vi "FindNodeByID.vi"(8 "error in (no error)":errorcluster, 9 "Node ID":string="//rect", 10 "Node Name (exact)":string="//rect", 11 "ParseSVG in":refnum<class "ParseSVG.lvclass">) -> (0 "error out":errorcluster, 2 "ID Match Node":refnum<k20>, 3 "ParseSVG out":refnum<class "ParseSVG.lvclass">)   [LabVIEW 2019, in "ParseSVG.lvclass"]
uses:
  ParseSVG.lvclass
  <vilib>/xml/NI_XML.lvlib
  <vilib>/xml/Close Reference(Node).vi
  <resource>/objmgr/DOMUserDefRef.rc
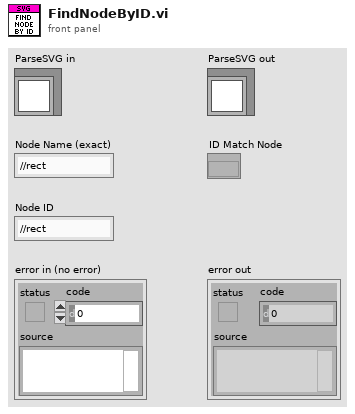
[diagram p1: front panel]
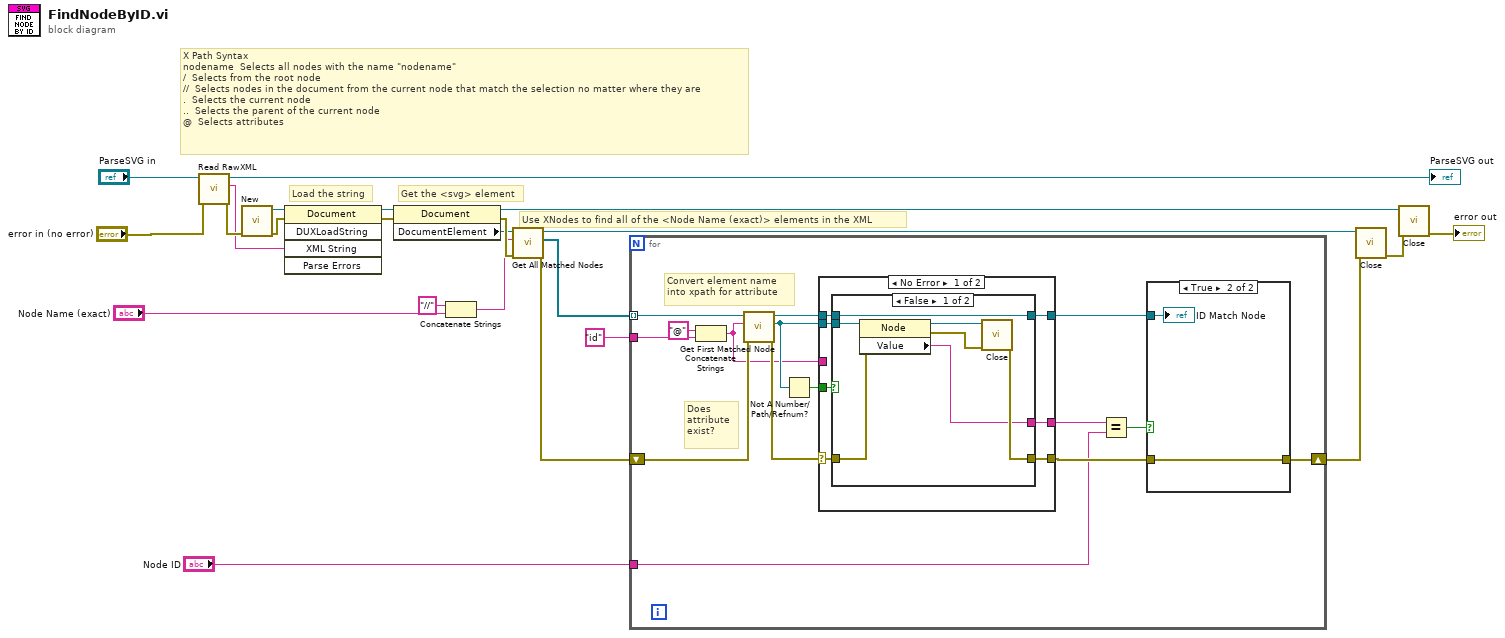
[diagram p0: block diagram]
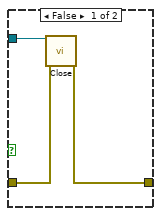
[diagram p2: hidden frame]
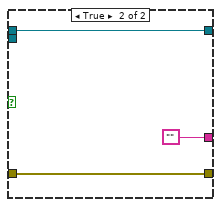
[diagram p3: hidden frame]
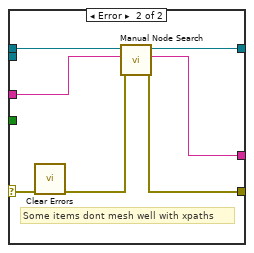
[diagram p4: hidden frame]
diagram:
  # "X Path Syntax\nnodename \tSelects all nodes with the name \"nodename\"\n/ \tSelects from the root node\n// \tSelects nodes in the document from the current node that match the selection no matter where they are\n. \tSelects the current node\n.. \tSelects the parent of the current node\n@ \tSelects attributes"
  # "Use XNodes to find all of the <Node Name (exact)> elements in the XML"
  # "Get the <svg> element"
  # "Load the string"
  n1 = call "Read RawXML.vi"("error in (no error)"="error in (no error)", "ParseXML in"="ParseSVG in") -> ("error out"=w22:errorcluster, "RawXML"=w8:string, "ParseXML out"=→"ParseSVG out":refnum<class "ParseSVG.lvclass">)  [unwired: 7 in]
  n2 = call <vilib>:"New.vi"("error in (no error)"=w22) -> ("error out"=w21:errorcluster, "DOM document out"=w17:refnum<k20>)  [unwired: 7 in]
  n3 = invoke class="Document" method="DUXLoadString"(reference=w17, error in=w21, "XML String"=w8) -> (reference out=w16:refnum<k20>, error out=w20:errorcluster)  [unwired: 2 in, 3 out]
  n4 = property class="Document"(reference=w16, error in=w20) -> (reference out=w15:refnum<k20>, error out=w19:errorcluster, "DocumentElement"=w14:refnum<k20>)
  n5 = Concatenate Strings("//" ("string"), "Node Name (exact)") -> (w10:string)
  n6 = call <vilib>:"Get All Matched Nodes.vi"("error in (no error)"=w19, "XPath expression"=w10, "node in"=w14) -> ("error out"=w2:errorcluster, "node result array"=w12:refnum<k20>[], "node out"=w13:refnum<k20>)  [unwired: 6 in]
  n7 = for {
    tunnel: w12 -> [w36] mode=indexing
    shift-right: [w34] -> w23
    shift-left: w2 -> [w37]
    tunnel: "id" -> [w33]
    tunnel: "Node ID" -> [w25]
    # "Convert element name into xpath for attribute"
    # "Does attribute exist?"
    n8 = Concatenate Strings("@" ("string"), w33) -> (w27:string)
    n9 = call <vilib>:"Get First Matched Node.vi"("error in (no error)"=w37, "XPath expression"=w27, "node in"=w36) -> ("error out"=w32:errorcluster, "node result"=w31:refnum<k20>, "node out"=w29:refnum<k20>)  [unwired: 6 in]
    n10 = Not A Number/Path/Refnum?(number/path/refnum=w31) -> (NaN/Path/Refnum?=w30:bool)
    n11 = case shown="No Error" w32 {
      selector: w32 -> [w49 w66]
      tunnel: [w50 w67] -> w38
      tunnel: w31 -> [w48 _]
      tunnel: w30 -> [w47 _]
      tunnel: w29 -> [w46 w63]
      tunnel: [w45 w64] -> w35
      tunnel: [w44 w61] -> w26
      tunnel: w27 -> [_ w62]
      frame No Error {
        n12 = case shown="False" w47 {
          tunnel: w49 -> [w57 w60]
          tunnel: [w56 w60] -> w50
          tunnel: w48 -> [w54 _]
          tunnel: w46 -> [w53 w59]
          tunnel: [w53 w59] -> w45
          tunnel: [w52 ""] -> w44
          frame False {
            n13 = property class="Node"(reference=w54, error in=w57) -> (reference out=w55:refnum<k20>, error out=w51:errorcluster, "Value"=w52:string)
            n14 = call-poly <vilib>:"Close.vi"("error in (no error)"=w51, "node"=w55) -> ("error out"=w56:errorcluster)  [unwired: 7 in]
          }
          frame True {
          }
        }
      }
      frame Error {
        # "Some items dont mesh well with xpaths"
        n15 = call <vilib>:"Clear Errors.vi"("error in (no error)"=w66) -> ("error out"=w65:errorcluster)  [unwired: 5 in, 1 out]
        n16 = call "Manual Node Search.vi"("error in (no error)"=w65, "XPath Syntax"=w62, "Node in"=w63) -> ("error out"=w67:errorcluster, "Value"=w61:string, "Node out"=w64:refnum<k20>)  [unwired: 6 in]
      }
    }
    n17 = Equal?(x=w26, y=w25) -> (x = y?=w24:bool)
    n18 = case shown="True" w24 {
      tunnel: w38 -> [w40 w43]
      tunnel: w35 -> [w41 w42]
      tunnel: [w39 w43] -> w34
      frame False {
        n19 = call-poly <vilib>:"Close.vi"("error in (no error)"=w40, "node"=w41) -> ("error out"=w39:errorcluster)  [unwired: 7 in]
      }
      frame True {
        "ID Match Node" <- w42
      }
    }
  }
  n20 = call-poly <vilib>:"Close.vi"("error in (no error)"=w23, "node"=w13) -> ("error out"=w18:errorcluster)  [unwired: 7 in]
  n21 = call-poly <vilib>:"Close.vi"("error in (no error)"=w18, "node"=w15) -> ("error out"=→"error out":errorcluster)  [unwired: 7 in]
